vi "SRV_Check Calculated Sensors Config.vi"(11 "All Sensors Config":T1[](array[typedef]) {"Register" format="%.0x"; "I2C Address" format="%.0x"; "Sample Period (ms)" min=10 max=60000 step=1; "Digital Mask" format="%.0x"; "Channel" format="%.0x"}) -> (1 "All OK?":bool, 2 "Error Message String":string)   [LabVIEW 2014]
uses:
  SRV_Sensor Config Cluster.ctl
  SRV_Sensor Analog-Digital.ctl
  SRV_Sensor Sampling Mode.ctl
  SRV_Sensor View Config Cluster.ctl
  SRV_Sensors Names.ctl
  SRV_Sensor PicoC Shared Var Type.ctl
  SRV_Sensor Number of Bytes.ctl
  SRV_Sensor Integer Word Type.ctl
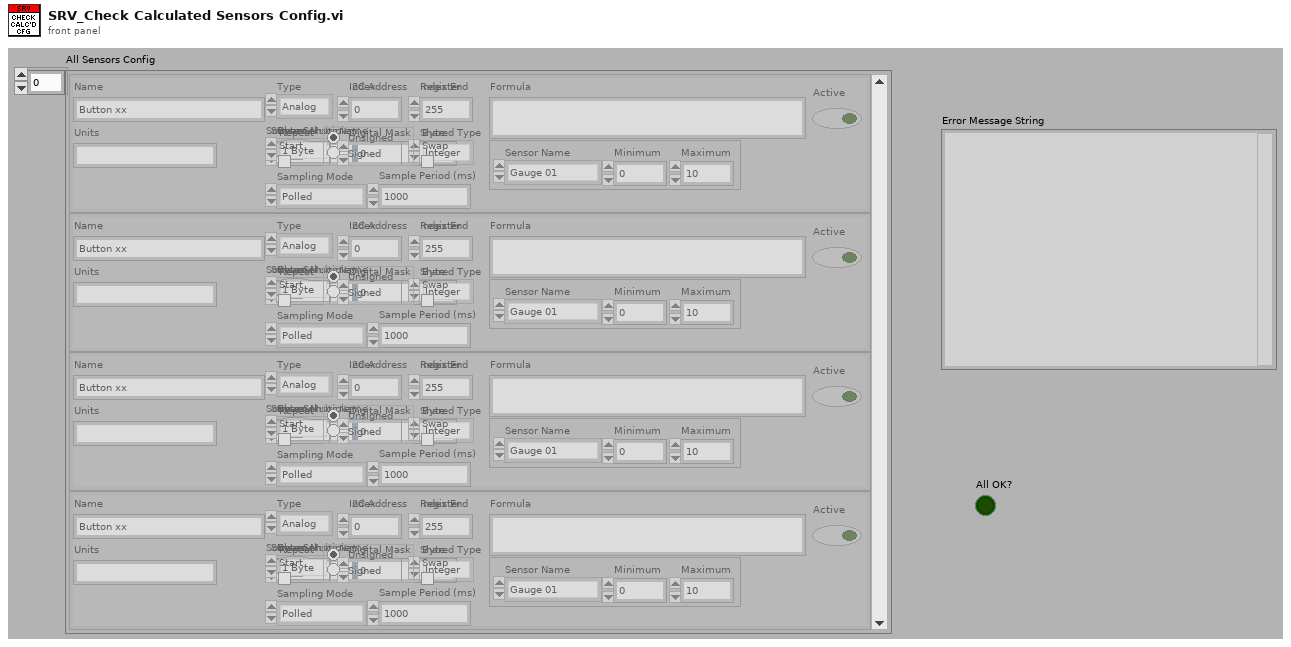
[diagram p1: front panel]
types:
  T1 = typedef "SRV_Sensor Config Cluster.ctl" = cluster{"Name":string, "A/D":T2, "I2C Address":u8, "Register":u8, "Channel":u8, "Digital Mask":u16, "Units":string, "Sampling Mode":T3, "Sample Period (ms)":u32, "Formula":string, "Sensor View Config":T4, "Active":bool, "PicoC Shared Var Type":T6, "Index":u8, "Stream Multiple?":bool, "Index End":u8, "Bytes":T7, "Source Sensor Name":string, "Repeat Start":bool, "Integer Word Type":T8, "Byte Swap":bool}
  T2 = typedef "SRV_Sensor Analog-Digital.ctl" = enum16{"Digital", "Analog", "PicoC Shared", "Calculated"}
  T3 = typedef "SRV_Sensor Sampling Mode.ctl" = enum16{"Polled", "Streaming"}
  T4 = typedef "SRV_Sensor View Config Cluster.ctl" = cluster{"Sensor Name":T5, "Minimum":dbl, "Maximum":dbl}
  T5 = typedef "SRV_Sensors Names.ctl" = enum16{"Gauge 01", "Gauge 02", "Gauge 03", "Gauge 04", "Meter 01", "Meter 02", "Meter 03", "Meter 04", "Numeric 01", "Numeric 02", "Numeric 03", "Numeric 04", "Numeric 05", "Numeric 06", "Numeric 07", "Numeric 08", "Boolean 01", "Boolean 02", "Boolean 03", "Boolean 04", "Boolean 05", "Boolean 06", "Boolean 07", "Boolean 08", "Boolean 09", "Boolean 10", "Boolean 11", "Boolean 12", "Boolean 13", "Boolean 14", "Boolean 15", "Boolean 16", "Boolean 17", "Boolean 18", "Boolean 19", "Boolean 20", "Boolean 21", "Boolean 22", "Boolean 23", "Boolean 24", "Boolean 25", "Boolean 26", "Boolean 27", "Boolean 28", "Boolean 29", "Boolean 30", "Boolean 31", "Boolean 32"}
  T6 = typedef "SRV_Sensor PicoC Shared Var Type.ctl" = enum16{"String", "Integer", "Float"}
  T7 = typedef "SRV_Sensor Number of Bytes.ctl" = enum16{"1 Byte", "2 Bytes"}
  T8 = typedef "SRV_Sensor Integer Word Type.ctl" = enum32{"Unsigned", "Signed"}
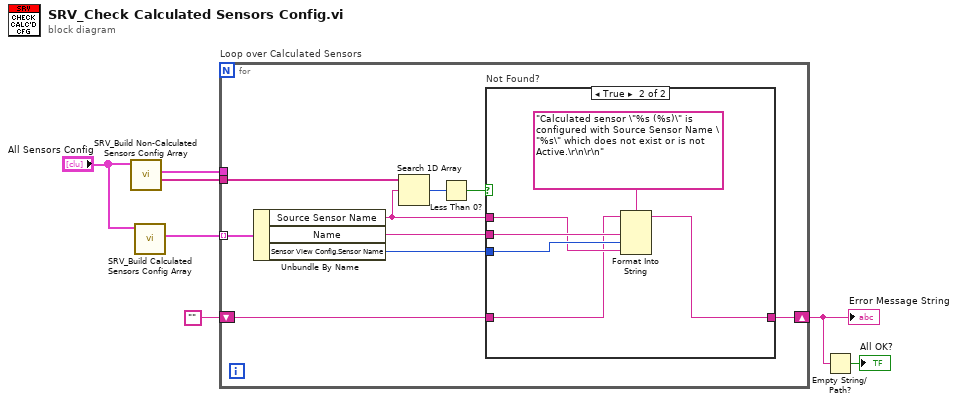
[diagram p0: block diagram]
diagram:
  n1 = call "SRV_Build Non-Calculated Sensors Config Array.vi"("Sensors Config"="All Sensors Config") -> ("Non-Calculated Sensors Names"=w4:string[], "Non-Calculated Sensors Config"=w5:T1[])  [unwired: 9 in]
  n2 = call "SRV_Build Calculated Sensors Config Array.vi"("Sensors Config"="All Sensors Config") -> ("Calculated Sensors Config"=w7:T1[])  [unwired: 10 in]
  n3 = for "Loop over Calculated Sensors" {
    tunnel: w7 -> [w16] mode=indexing
    tunnel: w5 -> [_]
    tunnel: w4 -> [w15]
    shift-right: [w8] -> w2
    shift-left: "" -> [w9]
    n4 = Unbundle By Name(w16) -> ("Source Sensor Name"=w10:string, "Name"=w12:string, "Sensor View Config.Sensor Name"=w11:T5)
    n5 = Search 1D Array(1D array=w15, element=w10) -> (index of element=w14:i32)  [unwired: 1 in]
    n6 = Less Than 0?(x=w14) -> (x < 0?=w13:bool)
    n7 = case "Not Found?" shown="True" w13 {
      tunnel: w12 -> [_ w22]
      tunnel: w11 -> [_ w21]
      tunnel: w10 -> [_ w20]
      tunnel: w9 -> [w17 w19]
      tunnel: [w17 w18] -> w8
      frame False {
      }
      frame True {
        n8 = Format Into String(format string="Calculated sensor \"%s (%s)\" is configured with Source Sensor Name \"%s\" which does not exist or is not Active.\r\n\r\n", initial string=w19, w22, w21, w20) -> (resulting string=w18:string)  [unwired: 1 in, 1 out]
      }
    }
  }
  "Error Message String" <- w2
  n9 = Empty String/Path?(string/path=w2) -> (empty?=→"All OK?":bool)
